vi "10-1.vi"() -> ()   [LabVIEW 2019, in "10.lvlib"]
uses:
  10.lvlib
panel:
  out "sum":i32
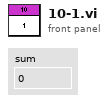
[diagram p1: front panel]
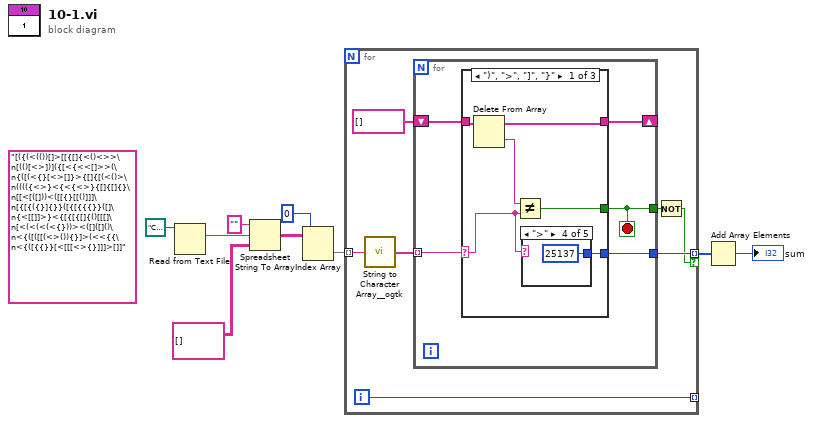
[diagram p0: block diagram]
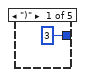
[diagram p2: hidden frame]
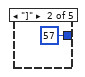
[diagram p3: hidden frame]
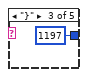
[diagram p4: hidden frame]
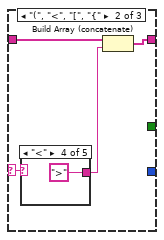
[diagram p6: hidden frame]
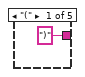
[diagram p7: hidden frame]
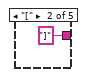
[diagram p8: hidden frame]
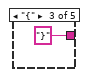
[diagram p9: hidden frame]
diagram:
  (unwired) "[({(<(())[]>[[{[]{<()<>>\n[(()[<>])]({[<{<<[]>>(\n{([(<{}[<>[]}>{[]{[(<()>\n(((({<>}<{<{<>}{[]{[]{}\n[[<[([]))<([[{}[[()]]]\n[{[{({}]{}}([{[{{{}}([]\n{<[[]]>}<{[{[{[]{()[[[]\n[<(<(<(<{}))><([]([]()\n<{([([[(<>()){}]>(<<{{\n<{([{{}}[<[[[<>{}]]]>[]]"
  n1 = Read from Text File(file (use dialog)=path "C:/Users/craig.walker/Documents/GitHub/lv2019-Advent-of-Code-2021/10/input.txt") -> (text=w2:string)  [unwired: 3 in, 3 out]
  n2 = Spreadsheet String To Array(format string="", spreadsheet string=w2, array type (2D Dbl)=string[][] []) -> (array=w6:string[][])  [unwired: 1 in]
  n3 = Index Array(array=w6, index (col)=0 ("disabled index (col)")) -> (element=w7:string[])  [unwired: 1 in]
  n4 = for {
    tunnel: w7 -> [w16] mode=indexing
    tunnel: [w14] -> w4 mode=indexing if=w10
    tunnel: [w12] -> _ mode=indexing
    i -> [w12]
    n5 = call <userlib>:"String to Character Array__ogtk.vi"("Input String"=w16) -> ("Character Array"=w15:string[])
    n6 = for {
      tunnel: w15 -> [w21] mode=indexing
      tunnel: [w20] -> w13
      tunnel: [w19] -> w14
      shift-right: [w18] -> _
      shift-left: string[] [] -> [w17]
      stop <- w20 stop-if-true
      n7 = case shown="\")\", \">\", \"]\", \"}\"" w21 {
        selector: w21 -> [w22 w33 _]
        tunnel: [w24 _ _] -> w20
        tunnel: [w27 _ _] -> w19
        tunnel: [w25 w35 w40] -> w18
        tunnel: w17 -> [w26 w34 w40]
        frame ")", ">", "]", "}" {
          n8 = Delete From Array(array=w26) -> (deleted portion=w23:string, array with subset deleted=w25:string[])  [unwired: 2 in]
          n9 = Not Equal?(x=w23, y=w22) -> (x != y?=w24:bool)
          n10 = case shown="\">\"" w22 {
            tunnel: [3 ("]") 57 ("]") 1197 ("]") 25137 ("]") _] -> w27
            frame ")" {
            }
            frame "]" {
            }
            frame "}" {
            }
            frame ">" {
            }
            frame Default {
            }
          }
        }
        frame "(", "<", "[", "{" {
          n11 = case shown="\"<\"" w33 {
            tunnel: [")" ("]") "]" ("]") "}" ("]") ">" ("]") _] -> w32
            frame "(" {
            }
            frame "[" {
            }
            frame "{" {
            }
            frame "<" {
            }
            frame Default {
            }
          }
          n12 = Build Array (concatenate)(w34, w32) -> (w35:string[])
        }
        frame Default {
        }
      }
    }
    n13 = Not(x=w13) -> (.not. x?=w10:bool)
  }
  n14 = Add Array Elements(numeric array=w4) -> (sum=→"sum":i32)
